vi "SDI-12 Continuous Operations.vi"() -> ()   [LabVIEW 2015]
doc: "A general set of examples of the SDI-12 API for a generic sensor. A tab control separates each example, and contains the following examples:\n1. Read Single.\n2. Read Multiple.\n3. Acknowledge Active.\n4. Change Address.\n5. Address Query.\n6. Send Identification."
uses:
  <vilib>/Utility/file.llb/Write Delimited Spreadsheet (string).vi
  <vilib>/Utility/file.llb/Write Delimited Spreadsheet (DBL).vi
  SDI-12.lvlib
panel:
  out "Measurements Out":dbl[](array[numeric])
  out "Address Out":string="a" caption="sensor address out"
  out "Number of Measurements Out":i32
  in  "Measurement Type In (Normal)":i32(ring)=1 items=["Normal", "Concurrent", "Continuous"]
  out "Parameter Out":i32(ring) items=["0", "1", "2", "3", "4", "5", "6", "7", "8", "9"]
  in  "Parameter In (0)":i32(ring) items=["0", "1", "2", "3", "4", "5", "6", "7", "8", "9"]
  in  "CRC (False)":bool
  out "CRC Out":bool
  out "Measurement Type Out":i32(ring) items=["Normal", "Concurrent", "Continuous"]
  out "Time (s)":dbl
  in  "stop":bool
  out "counter":i32
  in  "Sensor Address In":string="b"
  out "start time":timestamp
  out "new file path (Not A Path if cancelled)":path
  in  "Save File":bool
  in  "file directory (dialog if empty)":path=path "D:/Cascade/Raw Data files"
  in  "index":i32
  out "Array":timestamp[](array[timestamp])
  out "Waveform Chart":dbl[](graph)
  in  "Error In (No Error)":errorcluster
  in  "RS232 Port In":refnum<visa-resource-name>="COM11"
  out "Error Out":errorcluster
  # "deg C"
  # "pH"
  # "specific conductance"
  # "salinity or TDS"
  # "DO % saturation"
  # "DO mg/L"
  # "ORP"
  # "depth"
  # "battery"
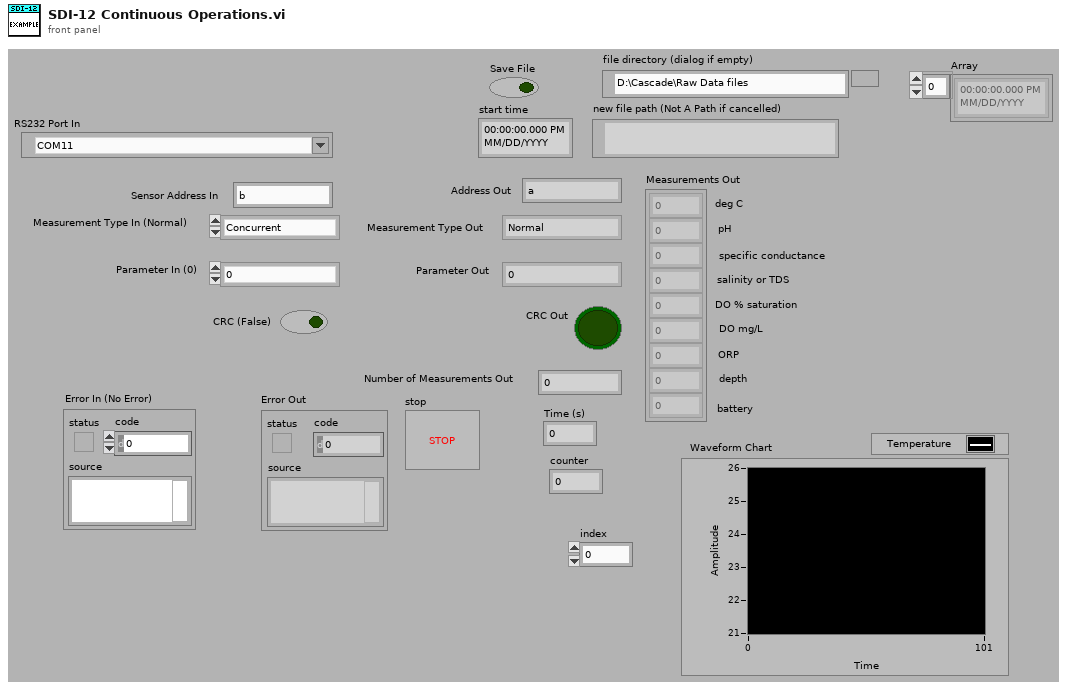
[diagram p1: front panel]
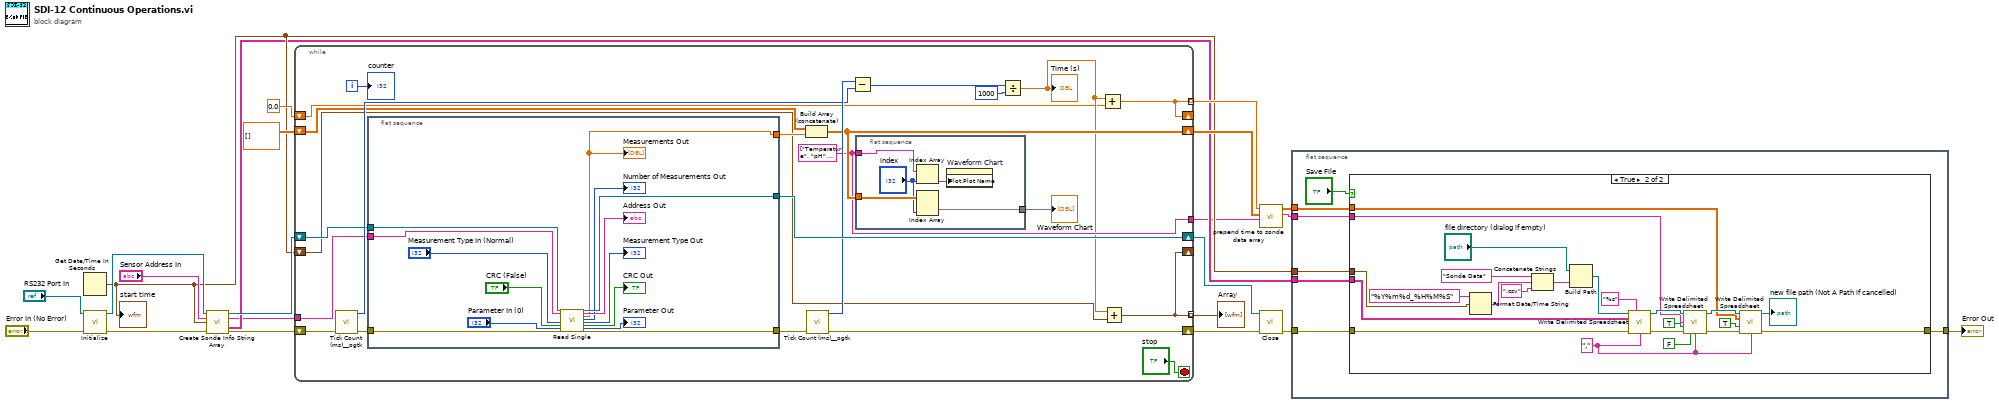
[diagram p0: block diagram]
diagram:
  n1 = Get Date/Time In Seconds() -> (seconds since 1Jan1904=w5:timestamp)
  "start time" <- w5
  n2 = call "Initialize.vi"("Error In (No Error)"="Error In (No Error)", "RS232 Port In"="RS232 Port In") -> ("Error Out"=w18:errorcluster, "RS232 Port Out"=w17:refnum<visa-resource-name>)  [unwired: 8 in]
  n3 = call "Create Sonde Info String Array.vi"("VISA Refnum in"=w17, "Sensor Address In"="Sensor Address In", "seconds since 1Jan1904"=w5, "error in (no error)"=w18) -> ("VISA Refnum out"=w16:refnum<visa-resource-name>, "Address Out"=w3:string, "Array"=w4:string[][], "error out"=w15:errorcluster)  [unwired: 8 in]
  n4 = while {
    shift-right: [w44] -> w19
    shift-left: w16 -> [w37]
    shift-right: [w45] -> w20
    shift-left: w15 -> [w36]
    shift-right: [w31] -> w11
    shift-left: dbl[][] [] -> [w32]
    tunnel: [w28] -> w13 mode=indexing
    shift-right: [w28] -> _
    shift-left: w5 -> [w29]
    tunnel: [w24] -> w12 mode=indexing
    tunnel: [w27] -> w2
    shift-right: [w24] -> _
    shift-left: 0.0 -> [w25]
    tunnel: w3 -> [w23]
    i -> [w34]
    stop <- "stop" stop-if-true
    w27 = string[] ["Temperature", "pH", "Specific Conductance", "Salinity", "DO % saturation", "DO", "ORP", "depth", "battery"] ("Measurement Labels")
    n5 = call <userlib>:"Tick Count (ms)__ogtk.vi"("error in (no error)"=w36) -> ("error out"=w42:errorcluster, "millisecond timer value"=w40:u32)  [unwired: 9 in]
    n6 = flat-sequence {
      tunnel: [w64] -> w44
      tunnel: [w63] -> w43
      tunnel: w42 -> [w54]
      tunnel: w37 -> [w53]
      tunnel: [w52] -> w33
      tunnel: w23 -> [w51]
      frame #0 {
        n7 = call "Read Single.vi"("RS232 Port In"=w53, "Sensor Address In"=w51, "Measurement Type In (Normal)"="Measurement Type In (Normal)", "CRC (False)"="CRC (False)", "Parameter In (0)"="Parameter In (0)", "Error In (No Error)"=w54) -> ("RS232 Port Out"=w64:refnum<visa-resource-name>, "Sensor Address Out"=→"Address Out":string, "Measurements Out"=w52:dbl[], "Number of Measurements Out"=→"Number of Measurements Out":i32, "Measurement Type Out"=→"Measurement Type Out":i32, "CRC Out"=→"CRC Out":bool, "Parameter Out"=→"Parameter Out":i32, "Error Out"=w63:errorcluster)  [unwired: 14 in]
        "Measurements Out" <- w52
      }
    }
    n8 = Build Array (concatenate)(w32, w33) -> (w31:dbl[][])
    n9 = call <userlib>:"Tick Count (ms)__ogtk.vi"("error in (no error)"=w43) -> ("error out"=w45:errorcluster, "millisecond timer value"=w41:u32)  [unwired: 9 in]
    n10 = Subtract(x=w41, y=w40) -> (x-y=w39:u32)
    n11 = flat-sequence {
      tunnel: w31 -> [w50]
      tunnel: [w49] -> w30
      tunnel: w27 -> [w48]
      frame #0 {
        n12 = Index Array(array=w48, index="index") -> (element=w46:string)
        n13 = Index Array(array=w50, index (col)="index") -> (element=w49:dbl[])  [unwired: 1 in]
        n14 = property on="Waveform Chart" class="WFChart (strict)"("Plot.Plot Name"=w46) -> ()  [unwired: 2 in, 2 out]
      }
    }
    n15 = Divide(x=w39, y=u32 1000) -> (x/y=w26:dbl)
    "Time (s)" <- w26
    n16 = Add(x=w26, y=w25) -> (x+y=w24:dbl)
    n17 = Add(x=w26, y=w29) -> (x+y=w28:timestamp)
    "counter" <- w34
    "Waveform Chart" <- w30
  }
  "Array" <- w13
  n18 = call "prepend time to sonde data array.vi"("Measurement Labels"=w2, "Sonde\nData Array"=w11, "Time Array"=w12) -> ("Header Array"=w1:string[], "Data Array"=w8:dbl[][])  [unwired: 7 in]
  n19 = call "Close.vi"("Error In (No Error)"=w20, "RS232 Port In"=w19) -> ("Error Out"=w10:errorcluster)  [unwired: 9 in]
  n20 = flat-sequence {
    tunnel: w10 -> [w71]
    tunnel: [w70] -> w9
    tunnel: w1 -> [w68]
    tunnel: w8 -> [w67]
    tunnel: w5 -> [w66]
    tunnel: w4 -> [w65]
    frame #0 {
      n21 = case shown="True" "Save File" {
        tunnel: [w72 w92] -> w70
        tunnel: w71 -> [w72 w77]
        tunnel: w68 -> [_ w73]
        tunnel: w67 -> [_ w90]
        tunnel: w66 -> [_ w84]
        tunnel: w65 -> [_ w75]
        frame False {
        }
        frame True {
          w74 = "," ("delimiter (\\t)")
          n22 = Format Date/Time String(time format string (%c)="%Y%m%d_%H%M%S", seconds (now)=w84) -> (date/time string=w83:string)  [unwired: 1 in]
          n23 = Concatenate Strings("Sonde Data" ("name or relative path"), w83, ".csv" ("string")) -> (w85:string)
          n24 = Build Path(base path="file directory (dialog if empty)", name or relative path=w85) -> (appended path=w80:path)
          n25 = call-poly <vilib>:"Write Delimited Spreadsheet.vi"("file path (dialog if empty)"=w80, "format (%s)"="%s" ("format (%.3f)"), "2D data"=w75, "error in (no error)"=w77, "delimiter (\\t)"=w74) -> ("new file path (Not A Path if cancelled)"=w79:path, "error out"=w76:errorcluster)  [unwired: 9 in]
          n26 = call-poly <vilib>:"Write Delimited Spreadsheet.vi"("file path (dialog if empty)"=w79, "1D data"=w73, "append to file? (F)"=TRUE, "error in (no error)"=w76, "transpose? (F)"=FALSE, "delimiter (\\t)"=w74) -> ("new file path (Not A Path if cancelled)"=w94:path, "error out"=w93:errorcluster)  [unwired: 8 in]
          n27 = call-poly <vilib>:"Write Delimited Spreadsheet.vi"("file path (dialog if empty)"=w94, "2D data"=w90, "append to file? (F)"=TRUE, "error in (no error)"=w93, "delimiter (\\t)"=w74) -> ("new file path (Not A Path if cancelled)"=→"new file path (Not A Path if cancelled)":path, "error out"=w92:errorcluster)  [unwired: 9 in]
        }
      }
    }
  }
  "Error Out" <- w9
